vi "Check for Duplicate Variables.vi"(7 "Command/Response Refnum in":T1 format="%.0x", 8 "error in (no error)":errorcluster, 11 "Command/Response Format in":string) -> (0 "error out":errorcluster, 2 "Variables":string[](array[string]), 3 "Command/Response Format out":string)   [LabVIEW 2018, in "Instrument Addon Scripting API.lvlib"]
uses:
  Instrument Addon Scripting API.lvlib
  <vilib>/NI Veristand/Custom Device API/Custom Device Item Ref.ctl
  <vilib>/NI Veristand/Custom Device API/Custom Device API.lvlib
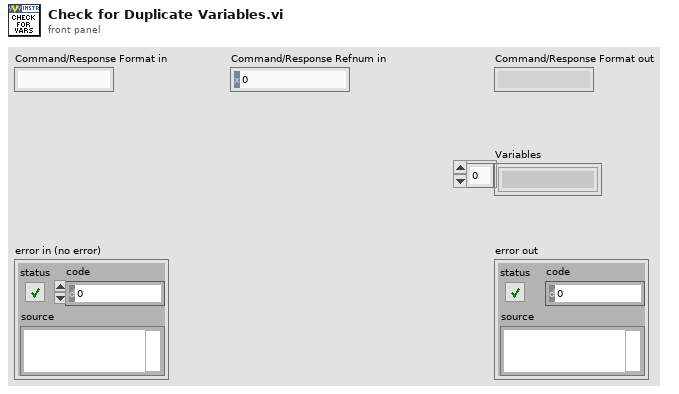
[diagram p1: front panel]
types:
  T1 = typedef "Custom Device API.lvlib/Custom Device Item Ref.ctl" = u64
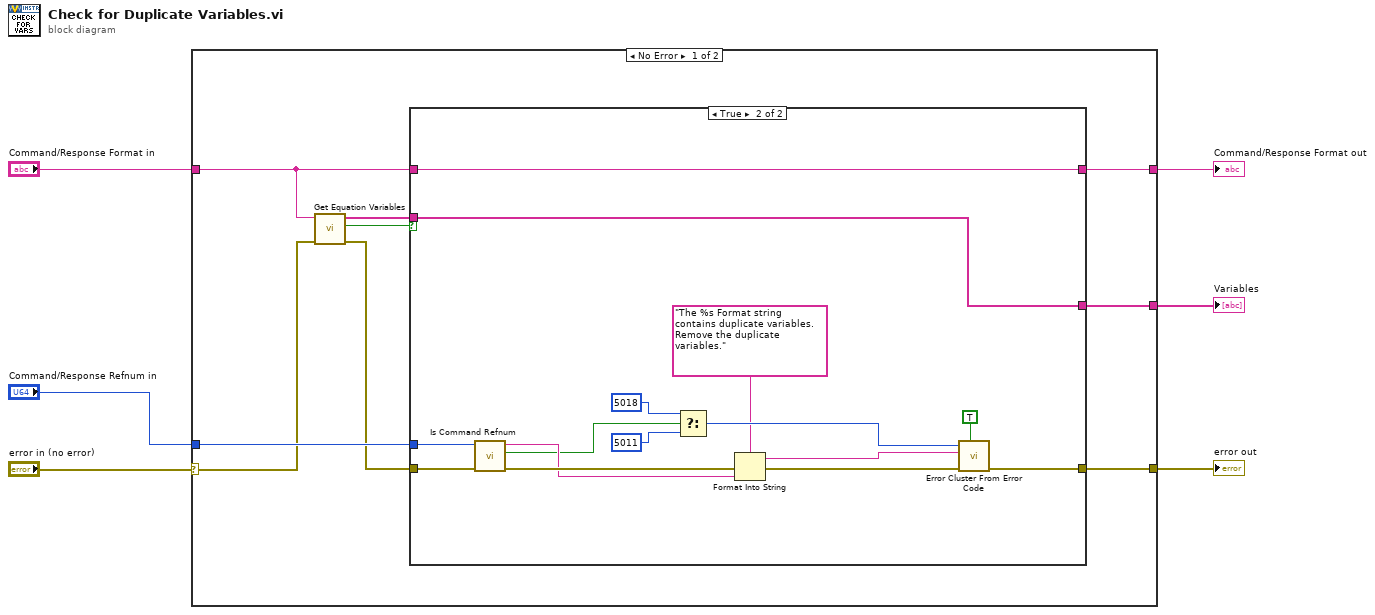
[diagram p0: block diagram]
diagram:
  n1 = case shown="No Error" "error in (no error)" {
    selector: "error in (no error)" -> [w10 w35]
    tunnel: [w15 w35] -> w6
    tunnel: [w14 _] -> w5
    tunnel: "Command/Response Format in" -> [w8 w34]
    tunnel: [w13 w34] -> w3
    tunnel: "Command/Response Refnum in" -> [w12 _]
    frame No Error {
      n2 = call "Get Equation Variables.vi"("error in (no error)"=w10, "Format String"=w8) -> ("error out"=w9:errorcluster, "Duplicate?"=w11:bool, "Variables out"=w7:string[])  [unwired: 7 in]
      n3 = case shown="True" w11 {
        tunnel: w9 -> [w18 w24]
        tunnel: [w18 w33] -> w15
        tunnel: w7 -> [w16 w32]
        tunnel: [w16 w32] -> w14
        tunnel: w8 -> [w17 w31]
        tunnel: [w17 w31] -> w13
        tunnel: w12 -> [_ w21]
        frame False {
        }
        frame True {
          n4 = call "Is Command Refnum.vi"("error in (no error)"=w24, "Command/Response Refnum in"=w21) -> ("error out"=w23:errorcluster, "Is Command?"=w20:bool, "Command/Response out"=w22:string)  [unwired: 7 in]
          n5 = Select(t=5018 ("error code (0)"), s=w20, f=5011 ("error code (0)")) -> (s? t:f=w27:i32)
          n6 = Format Into String(format string="The %s Format string contains duplicate variables. Remove the duplicate variables." ("error message (\"\")"), error in=w23, w22) -> (resulting string=w26:string, error out=w28:errorcluster)  [unwired: 1 in]
          n7 = call <vilib>:"Error Cluster From Error Code.vi"("show call chain? (False)"=TRUE, "error in (no error)"=w28, "error message (\"\")"=w26, "error code (0)"=w27) -> ("error out"=w33:errorcluster)  [unwired: 5 in]
        }
      }
    }
    frame Error {
    }
  }
  "error out" <- w6
  "Variables" <- w5
  "Command/Response Format out" <- w3
